vi "OPC UA Client-Write.vi"() -> ()   [LabVIEW 2018]
uses:
  <vilib>/OPCUA/controls/Write Variant Request.ctl
  <vilib>/OPCUA/controls/NodeId.ctl
  <vilib>/OPCUA/controls/Write Status.ctl
  <vilib>/OPCUA/client/Multiple Write Variant.vi
  <vilib>/OPCUA/NI OPC UA Client.lvlib
panel:
  in  "Node Id":string="ns=2;s=ProcessData.Temperature"
  in  "Stop Button":bool
  in  "Temperature Value":dbl=22.0
  in  "Server Endpoint URL":string="opc.tcp://XPS15HPH:49580"
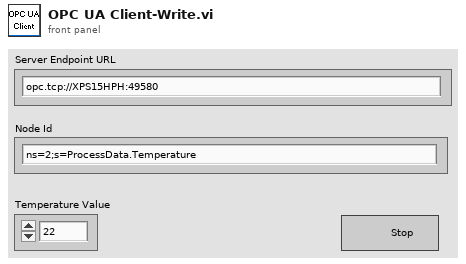
[diagram p1: front panel]
types:
  T1 = cluster{"message mode":enum16{"None", "Sign", "Sign and Encrypt"}, "security":enum16{"Basic256", "Basic128Rsa15"}}
  T2 = typedef "OPC UA Client Refnum.ctl" = refnum<k21>
  T3 = typedef "Write Variant Request.ctl" = cluster{"node ID":T4, "value":variant, "timestamp (current time)":timestamp, "node status":T5}
  T4 = typedef "NodeId.ctl" = string
  T5 = typedef "Write Status.ctl" = u32
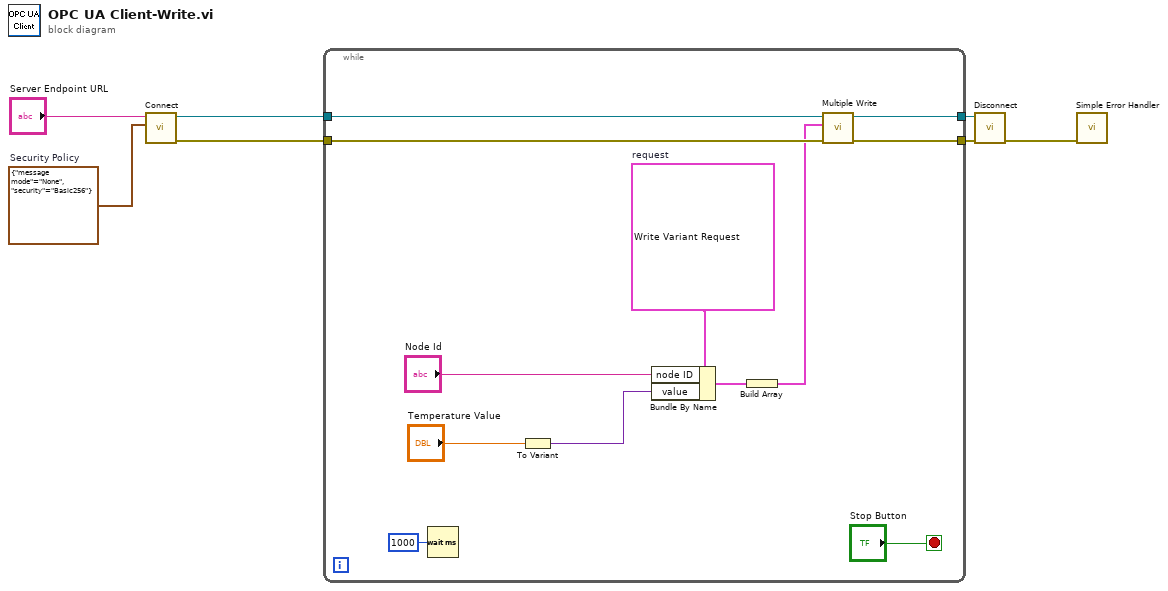
[diagram p0: block diagram]
diagram:
  w1 = T1 {"message mode"=enum."None", "security"=enum."Basic256"}  # Security Policy
  n1 = call <vilib>:"Connect.vi"("security policy"=w1, "server endpoint URL"="Server Endpoint URL") -> ("error out"=w6:errorcluster, "OPC UA client refnum out"=w7:T2)  [unwired: 7 in, 1 out]
  n2 = while {
    tunnel: w7 -> [w17]
    tunnel: w6 -> [w16]
    tunnel: [w15] -> w5
    tunnel: [w14] -> w3
    stop <- "Stop Button" stop-if-true
    w12 = T3 {"node ID"="", "value"=variant, "timestamp (current time)"=timestamp(0 s since 1904-01-01), "node status"=0}  # request
    n3 = Wait (ms)(milliseconds to wait=u32 1000) -> ()  [unwired: 1 out]
    n4 = To Variant(anything="Temperature Value") -> (Variant=w8:variant)
    n5 = Bundle By Name(cluster=w12, "node ID"="Node Id", "value"=w8) -> (w11:T3)
    n6 = Build Array(w11) -> (w10:T3[])
    n7 = call-poly <vilib>:"Multiple Write.vi"("error in (no error)"=w16, "requests"=w10, "OPC UA client refnum in"=w17) -> ("error out"=w14:errorcluster, "OPC UA client refnum out"=w15:T2)  [unwired: 5 in, 2 out]
  }
  n8 = call <vilib>:"Disconnect.vi"("error in (no error)"=w3, "OPC UA client refnum in"=w5) -> ("error out"=w4:errorcluster)  [unwired: 9 in]
  n9 = call <vilib>:"Simple Error Handler.vi"("error in (no error)"=w4) -> ()  [unwired: 4 in, 5 out]
